vi "Default Instrument Setup.vi"(8 "error in (no error)":errorcluster, 11 "VISA resource name":refnum<visa-resource-name>) -> (0 "error out":errorcluster, 3 "VISA resource name out":refnum<visa-resource-name>)   [LabVIEW 2020, in "Agilent 90000 Series.lvlib"]
doc: "This Utility VI sends a default command string to the instrument whenever a new VISA session is opened, or the instrument is reset. Use this VI as a subVI for the Initialize and Reset VIs. Altering this VI could cause these two VIs to operate incorrectly."
uses:
  Agilent 90000 Series.lvlib
  <vilib>/regexp/Match Regular Expression.xnode
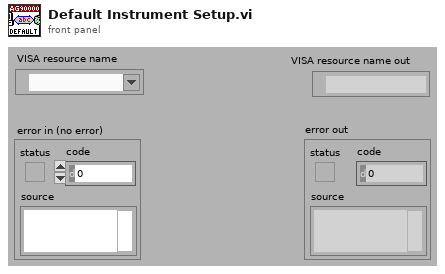
[diagram p1: front panel]
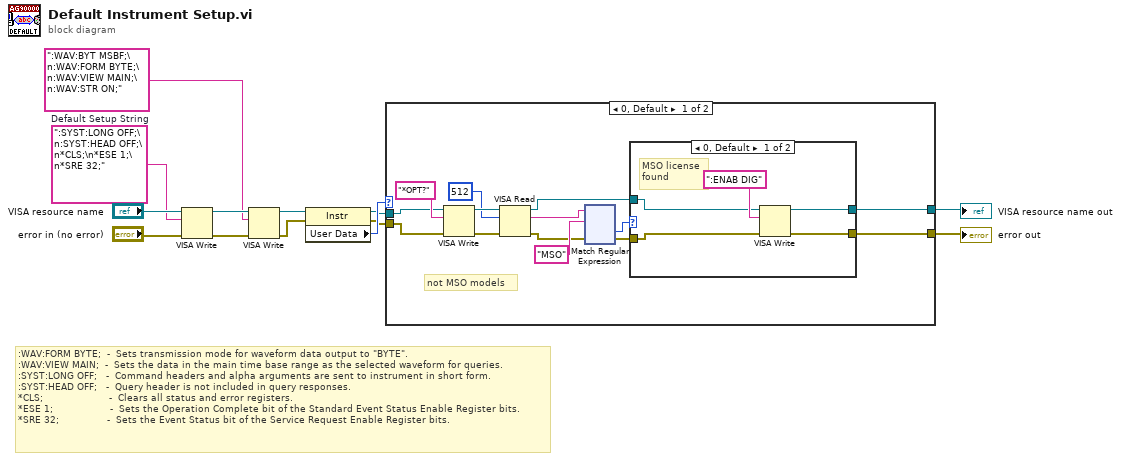
[diagram p0: block diagram]
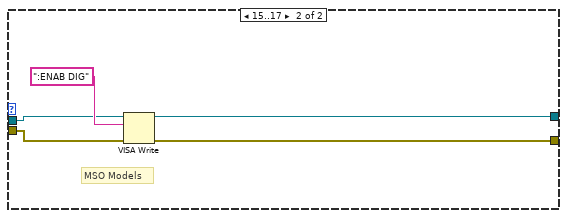
[diagram p3: hidden frame]
diagram:
  w11 = ":SYST:LONG OFF;\n:SYST:HEAD OFF;\n*CLS;\n*ESE 1;\n*SRE 32;"  # Default Setup String
  # ":WAV:FORM BYTE;  -  Sets transmission mode for waveform data output to \"BYTE\".\n:WAV:VIEW MAIN;  -  Sets the data in the main time base range as the selected waveform for queries.\n:SYST:LONG OFF;   -  Command headers and alpha arguments are sent to instrument in short form.\n:SYST:HEAD OFF;   -  Query header is not included in query responses.\n*CLS;                      -  Clears all status and error registers.\n*ESE 1;                   -  Sets the Operation Complete bit of the Standard Event Status Enable Register bits.\n*SRE 32;                -  Sets the Event Status bit of the Service Request Enable Register bits."
  n1 = VISA Write(VISA resource name="VISA resource name", write buffer=w11, error in (no error)="error in (no error)") -> (VISA resource name out=w10:refnum<visa-resource-name>, error out=w9:errorcluster)  [unwired: 1 out]
  n2 = VISA Write(VISA resource name=w10, write buffer=":WAV:BYT MSBF;\n:WAV:FORM BYTE;\n:WAV:VIEW MAIN;\n:WAV:STR ON;", error in (no error)=w9) -> (VISA resource name out=w7:refnum<visa-resource-name>, error out=w6:errorcluster)  [unwired: 1 out]
  n3 = property class="Instr"(reference=w7, error in=w6) -> (reference out=w4:refnum<visa-resource-name>, error out=w3:errorcluster, "User Data"=w5:u32)
  n4 = case shown="0, Default" w5 {
    tunnel: w4 -> [w26 w152]
    tunnel: w3 -> [w25 w151]
    tunnel: [w14 w150] -> w2
    tunnel: [w16 w149] -> w1
    frame 0, Default {
      # "not MSO models"
      n5 = VISA Write(VISA resource name=w26, write buffer="*OPT?", error in (no error)=w25) -> (VISA resource name out=w23:refnum<visa-resource-name>, error out=w24:errorcluster)  [unwired: 1 out]
      n6 = VISA Read(VISA resource name=w23, byte count=u32 512, error in (no error)=w24) -> (VISA resource name out=w15:refnum<visa-resource-name>, read buffer=w21:string, error out=w19:errorcluster)  [unwired: 1 out]
      n7 = xnode "Match Regular Expression"("input string"=w21, "regular expression"="MSO", "error in"=w19) -> ("offset past match"=w18:i32, "error out"=w17:errorcluster)  [unwired: 3 in, 3 out]
      n8 = case shown="0, Default" w18 {
        tunnel: w17 -> [w31 w33]
        tunnel: [w30 w33] -> w16
        tunnel: w15 -> [w29 w34]
        tunnel: [w28 w34] -> w14
        frame 0, Default {
          # "MSO license\nfound"
          n9 = VISA Write(VISA resource name=w29, write buffer=":ENAB DIG", error in (no error)=w31) -> (VISA resource name out=w28:refnum<visa-resource-name>, error out=w30:errorcluster)  [unwired: 1 out]
        }
        frame -1 {
          # "not found"
        }
      }
    }
    frame 15..17 {
      # "MSO Models"
      n10 = VISA Write(VISA resource name=w152, write buffer=":ENAB DIG", error in (no error)=w151) -> (VISA resource name out=w150:refnum<visa-resource-name>, error out=w149:errorcluster)  [unwired: 1 out]
    }
  }
  "error out" <- w1
  "VISA resource name out" <- w2
